vi "Mandelbrot V2.vi"() -> ()   [LabVIEW 2011]
panel:
  out "Ymax":dbl
  out "Ymin":dbl
  out "Xmax":dbl
  out "Xmin":dbl
  in  "Default":bool
  out "Duration (S)":dbl
  out "End Time":timestamp
  out "Start Time":timestamp
  out "C":cdb
  out "Intensity Graph":i32[][](graph)
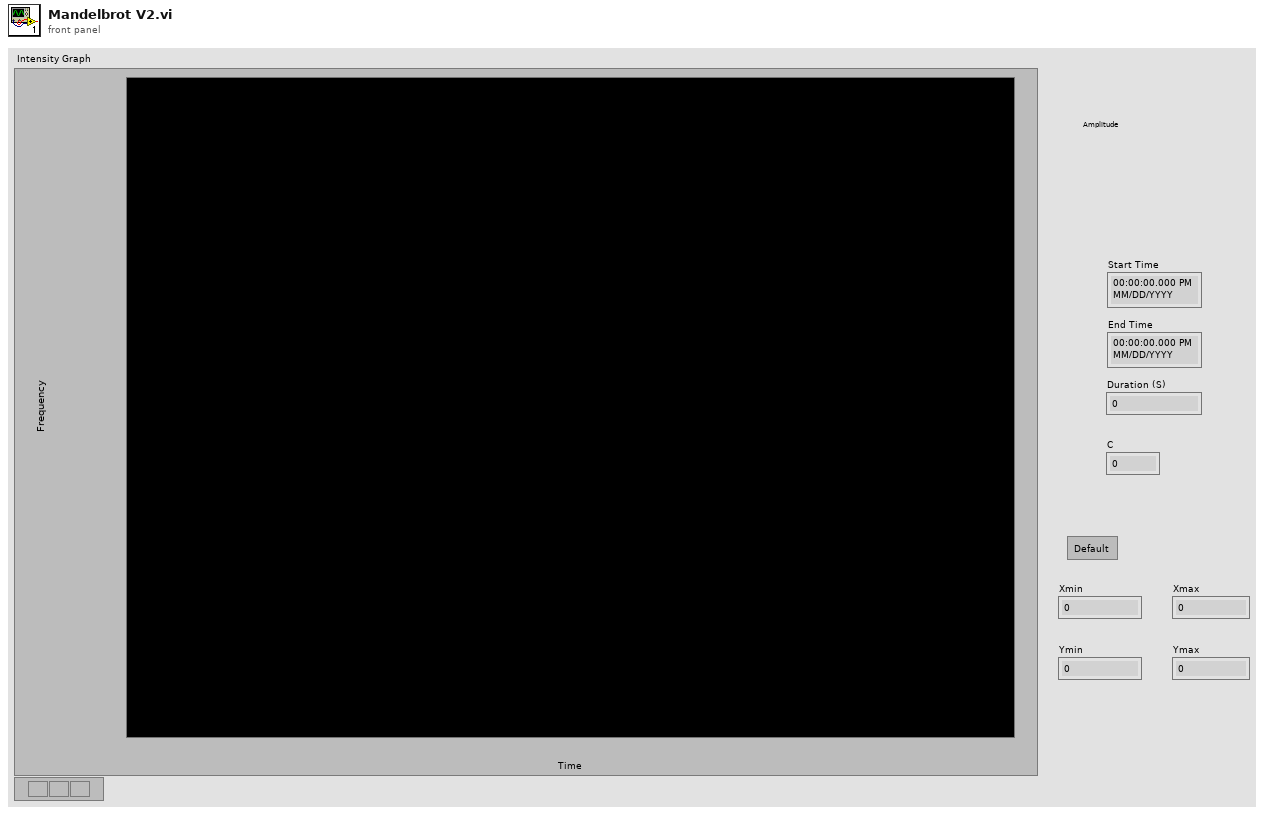
[diagram p1: front panel]
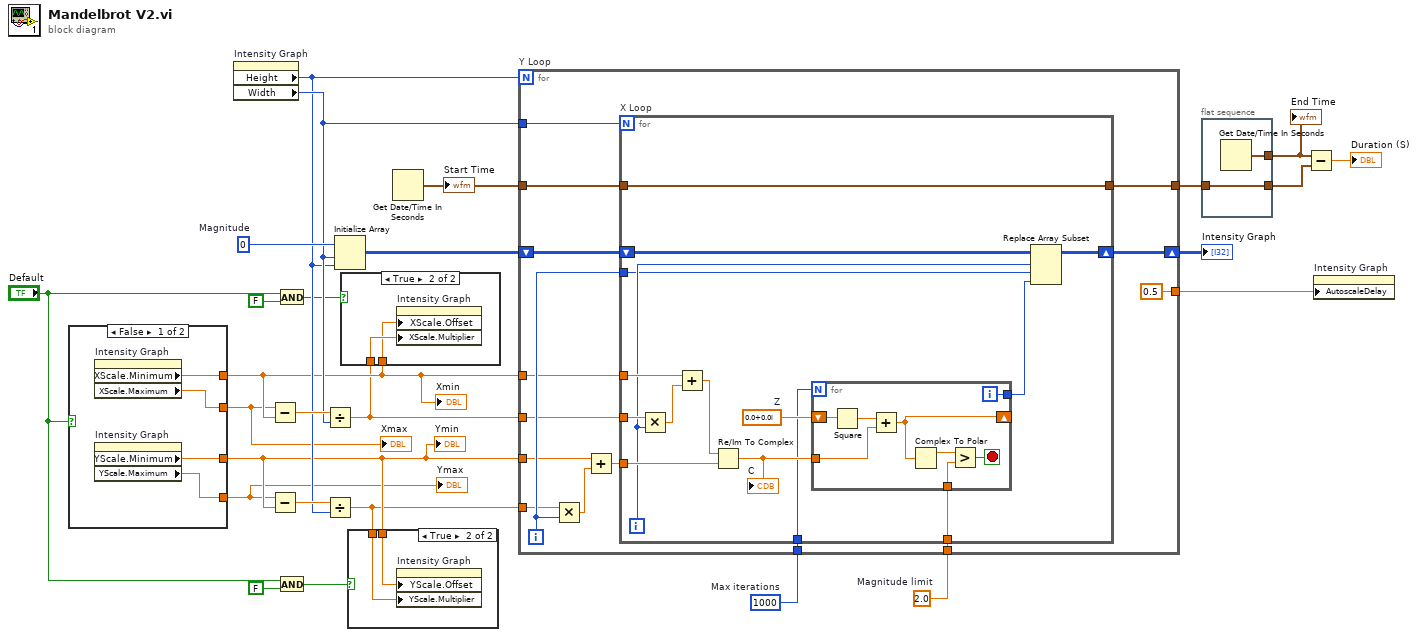
[diagram p0: block diagram]
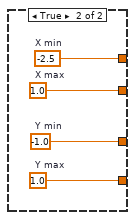
[diagram p4: hidden frame]
diagram:
  w21 = 2.0  # Magnitude limit
  w22 = 1000  # Max iterations
  w25 = 0  # Magnitude
  n1 = case shown="False" "Default" {
    tunnel: [w30 w34] -> w11
    tunnel: [w29 w33] -> w8
    tunnel: [w28 w32] -> w12
    tunnel: [w27 w31] -> w7
    frame False {
      n2 = property on="Intensity Graph" class="IntGraph (strict)"() -> ("XScale.Minimum"=w30:dbl, "XScale.Maximum"=w29:dbl)  [unwired: 2 in, 2 out]
      n3 = property on="Intensity Graph" class="IntGraph (strict)"() -> ("YScale.Minimum"=w28:dbl, "YScale.Maximum"=w27:dbl)  [unwired: 2 in, 2 out]
    }
    frame True {
      w32 = -1.0  # Y min
      w31 = 1.0  # Y max
      w34 = -2.5  # X min
      w33 = 1.0  # X max
    }
  }
  "Ymin" <- w12
  "Ymax" <- w7
  "Xmin" <- w11
  "Xmax" <- w8
  n4 = property on="Intensity Graph" class="IntGraph (strict)"() -> ("Height"=w14:u32, "Width"=w15:u32)  [unwired: 2 in, 2 out]
  n5 = Subtract(x=w8, y=w11) -> (x-y=w26:dbl)
  n6 = Subtract(x=w7, y=w12) -> (x-y=w23:dbl)
  n7 = And(x="Default", y=FALSE) -> (x .and. y?=w3:bool)
  n8 = And(x="Default", y=FALSE) -> (x .and. y?=w5:bool)
  n9 = Divide(x=w26, y=w15) -> (x/y=w9:dbl)
  n10 = Divide(x=w23, y=w14) -> (x/y=w10:dbl)
  n11 = Initialize Array(w25, w15, w14) -> (w24:i32[][])
  n12 = case shown="True" w3 {
    tunnel: w9 -> [_ w36]
    tunnel: w11 -> [_ w35]
    frame False {
    }
    frame True {
      n13 = property on="Intensity Graph" class="IntGraph (strict)"("XScale.Offset"=w35, "XScale.Multiplier"=w36) -> ()  [unwired: 2 in, 2 out]
    }
  }
  n14 = case shown="True" w5 {
    tunnel: w10 -> [_ w38]
    tunnel: w12 -> [_ w37]
    frame False {
    }
    frame True {
      n15 = property on="Intensity Graph" class="IntGraph (strict)"("YScale.Offset"=w37, "YScale.Multiplier"=w38) -> ()  [unwired: 2 in, 2 out]
    }
  }
  n16 = Get Date/Time In Seconds() -> (seconds since 1Jan1904=w20:timestamp)
  "Start Time" <- w20
  n17 = for "Y Loop" {
    N: w14 -> [_]
    tunnel: w9 -> [w46]
    tunnel: w11 -> [w48]
    shift-right: [w40] -> w13
    shift-left: w24 -> [w51]
    tunnel: w12 -> [w49]
    tunnel: w10 -> [w47]
    tunnel: w22 -> [w45]
    tunnel: w21 -> [w44]
    tunnel: w15 -> [w43]
    tunnel: w20 -> [w42]
    tunnel: [w41] -> w19
    tunnel: [sgl 0.5 ("Autoscale Delay")] -> w6
    i -> [w50]
    n18 = Multiply(x=w47, y=w50) -> (x*y=w53:dbl)
    n19 = Add(x=w49, y=w53) -> (x+y=w52:dbl)
    n20 = for "X Loop" {
      N: w43 -> [_]
      tunnel: w46 -> [w66]
      tunnel: w52 -> [w67]
      tunnel: w48 -> [w65]
      shift-right: [w61] -> w40
      shift-left: w51 -> [w62]
      tunnel: w50 -> [w56]
      tunnel: w45 -> [w59]
      tunnel: w44 -> [w58]
      tunnel: w42 -> [w55]
      tunnel: [w55] -> w41
      i -> [w57]
      w60 = cdb 0.0+0.0i  # Z
      n21 = Multiply(x=w66, y=w57) -> (x*y=w68:dbl)
      n22 = Add(x=w65, y=w68) -> (x+y=w64:dbl)
      n23 = Re/Im To Complex(1:w67, 2:w64) -> (0:w63:cdb)
      "C" <- w63
      n24 = for {
        N: w59 -> [_]
        tunnel: w63 -> [w75]
        shift-right: [w73] -> _
        shift-left: w60 -> [w76]
        tunnel: w58 -> [w71]
        tunnel: [w69] -> w54
        i -> [w69]
        stop <- w70 stop-if-true
        n25 = Square(x=w76) -> (x^2=w74:cdb)
        n26 = Add(x=w74, y=w75) -> (x+y=w73:cdb)
        n27 = Complex To Polar(r * e^(i*theta)=w73) -> (r=w72:dbl)  [unwired: 1 out]
        n28 = Greater?(x=w72, y=w71) -> (0:w70:bool)
      }
      n29 = Replace Array Subset(array=w62, new element=w54, index (row)=w57, index (col)=w56) -> (w61:i32[][])
    }
  }
  "Intensity Graph" <- w13
  n30 = flat-sequence {
    tunnel: w19 -> [w77]
    tunnel: [w78] -> w17
    tunnel: [w77] -> w18
    frame #0 {
      n31 = Get Date/Time In Seconds() -> (seconds since 1Jan1904=w78:timestamp)
    }
  }
  n32 = Subtract(x=w17, y=w18) -> (x-y=→"Duration (S)":dbl)
  n33 = property on="Intensity Graph" class="IntGraph (strict)"("AutoscaleDelay"=w6) -> ()  [unwired: 2 in, 2 out]
  "End Time" <- w17
